vi "Save Data.vi"(8 "error in (no error)":errorcluster, 11 "Data":waveform(dbl)[](array[waveform])) -> (0 "error out":errorcluster)   [LabVIEW 2017]
doc: "Saves data to disk."
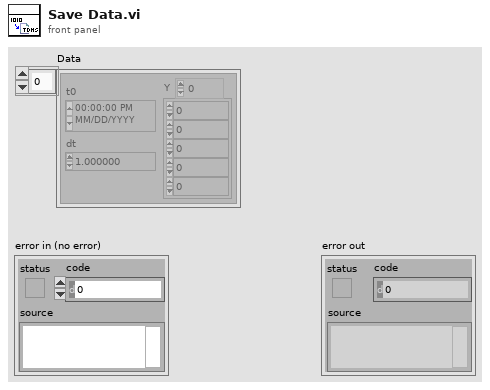
[diagram p1: front panel]
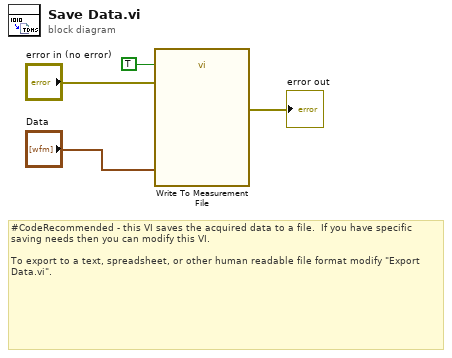
[diagram p0: block diagram]
diagram:
  # "#CodeRecommended - this VI saves the acquired data to a file.  If you have specific saving needs then you can modify this VI.\n\nTo export to a text, spreadsheet, or other human readable file format modify \"Export Data.vi\"."
  n1 = call "Write To Measurement File"("Signals"="Data", "Reset"=TRUE, "error in (no error)"="error in (no error)") -> ("error out"=→"error out":errorcluster)  [unwired: 14 in, 2 out]
